vi "frw_csv2array.vi"(8 "error in":errorcluster, 11 "file path":path) -> (0 "error out":errorcluster, 1 "values":dbl[][](array[numeric]), 2 "tags":string, 3 "headerarray":string[](array[string]))   [LabVIEW 2013]
doc: "Reas a CSV file and put the data in a 2D array"
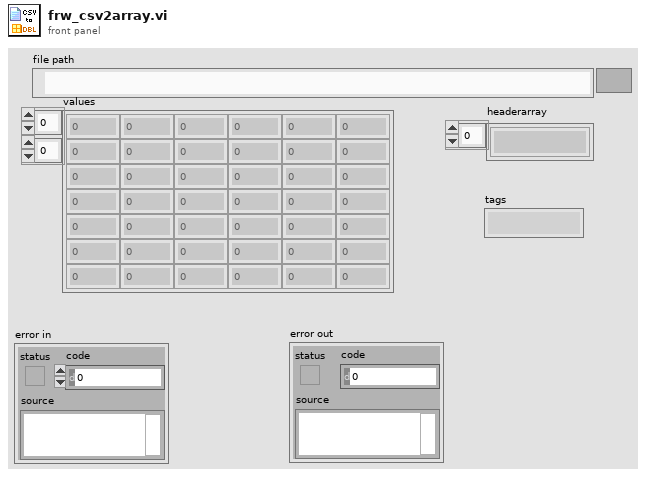
[diagram p1: front panel]
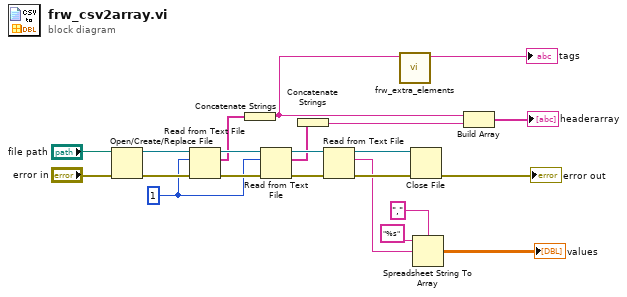
[diagram p0: block diagram]
diagram:
  w13 = 1 ("count")
  n1 = Open/Create/Replace File(file path (use dialog)="file path", error in="error in") -> (refnum out=w20:refnum<file>, error out=w19:errorcluster)  [unwired: 4 in, 1 out]
  n2 = Read from Text File(file (use dialog)=w20, count=w13, error in=w19) -> (refnum out=w14:refnum<file>, text=w3:string[], error out=w15:errorcluster)  [unwired: 1 in, 1 out]
  n3 = Concatenate Strings(w3) -> (w2:string)
  n4 = Read from Text File(file (use dialog)=w14, count=w13, error in=w15) -> (refnum out=w11:refnum<file>, text=w7:string[], error out=w12:errorcluster)  [unwired: 1 in, 1 out]
  n5 = Concatenate Strings(w7) -> (w6:string)
  n6 = Read from Text File(file (use dialog)=w11, error in=w12) -> (refnum out=w9:refnum<file>, text=w8:string, error out=w10:errorcluster)  [unwired: 2 in, 1 out]
  n7 = call "frw_extra_elements.vi"("string"=w2) -> ("data_format"=→"tags":string)  [unwired: 6 in, 4 out]
  n8 = Close File(refnum=w9, error in=w10) -> (error out=→"error out":errorcluster)  [unwired: 1 out]
  n9 = Spreadsheet String To Array(delimiter (Tab)=",", format string="%s", spreadsheet string=w8) -> (array=→"values":dbl[][])  [unwired: 1 in]
  n10 = Build Array(w2, w6) -> (→"headerarray":string[])
